vi "Ref Elevator Position.vi"(8 "error in (no error)":errorcluster, 11 "Sim Sensor Interface in":refnum<class "Sim Sensor Interface.lvclass">) -> (0 "error out":errorcluster, 2 "Elevator Position":refnum<vi>, 3 "Sim Sensor Interface out":refnum<class "Sim Sensor Interface.lvclass">)   [LabVIEW 2019, in "Simulated Sensor Interface Actor.lvlib" / "Sim Sensor Interface.lvclass"]
uses:
  Sim Sensor Interface.lvclass
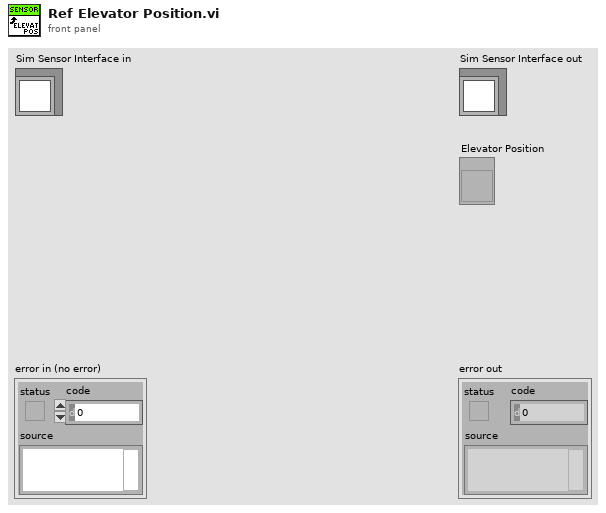
[diagram p1: front panel]
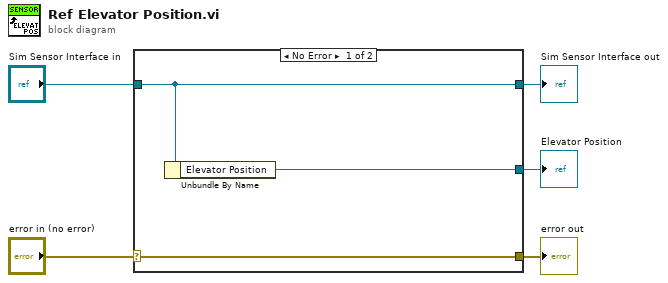
[diagram p0: block diagram]
diagram:
  n1 = case shown="No Error" "error in (no error)" {
    selector: "error in (no error)" -> [w8 w9]
    tunnel: [w8 w9] -> w4
    tunnel: [w7 w10] -> w2
    tunnel: "Sim Sensor Interface in" -> [w7 w10]
    tunnel: [w6 _] -> w1
    frame No Error {
      n2 = Unbundle By Name(w7) -> ("Elevator Position"=w6:refnum<vi>)
    }
    frame Error {
    }
  }
  "error out" <- w4
  "Sim Sensor Interface out" <- w2
  "Elevator Position" <- w1
